vi "gl_Initialise_Images.vi"() -> (3 "Live image refs":T1)   [LabVIEW 2017]
uses:
  User Interface/Queue/Live graphs queue/Typedefs/Live imaging queue element.ctl
  <vilib>/vision/Image Controls.llb/IMAQ Image.ctl
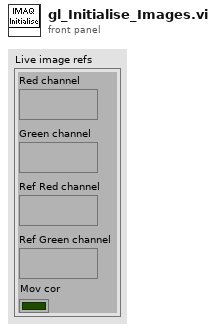
[diagram p1: front panel]
types:
  T1 = typedef "Live imaging queue element.ctl" = cluster{"Red channel":T2, "Green channel":T2, "Ref Red channel":T2, "Ref Green channel":T2, "Mov cor":bool}
  T2 = typedef "IMAQ Image.ctl" = refnum<image>
  T3 = typedef "Image Type" = u32
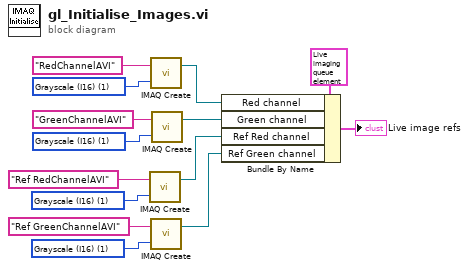
[diagram p0: block diagram]
diagram:
  w3 = T3 1 items=["Grayscale (U8)", "Grayscale (I16)", "Grayscale (SGL)", "Complex (CSG)", "RGB (U32)", "HSL (U32)", "RGB (U64)", "Grayscale (U16)"] ("Image Type")
  w6 = T3 1 items=["Grayscale (U8)", "Grayscale (I16)", "Grayscale (SGL)", "Complex (CSG)", "RGB (U32)", "HSL (U32)", "RGB (U64)", "Grayscale (U16)"] ("Image Type")
  w14 = T3 1 items=["Grayscale (U8)", "Grayscale (I16)", "Grayscale (SGL)", "Complex (CSG)", "RGB (U32)", "HSL (U32)", "RGB (U64)", "Grayscale (U16)"] ("Image Type")
  w11 = T3 1 items=["Grayscale (U8)", "Grayscale (I16)", "Grayscale (SGL)", "Complex (CSG)", "RGB (U32)", "HSL (U32)", "RGB (U64)", "Grayscale (U16)"] ("Image Type")
  n1 = call "IMAQ Create"("Image Name"="Ref RedChannelAVI", "Image Type"=w3) -> ("New Image"=w2:T2)  [unwired: 3 in, 1 out]
  n2 = call "IMAQ Create"("Image Name"="RedChannelAVI", "Image Type"=w14) -> ("New Image"=w9:T2)  [unwired: 3 in, 1 out]
  n3 = call "IMAQ Create"("Image Name"="Ref GreenChannelAVI", "Image Type"=w6) -> ("New Image"=w1:T2)  [unwired: 3 in, 1 out]
  n4 = call "IMAQ Create"("Image Name"="GreenChannelAVI", "Image Type"=w11) -> ("New Image"=w8:T2)  [unwired: 3 in, 1 out]
  n5 = Bundle By Name(cluster=T1 {"Red channel"=refnum, "Green channel"=refnum, "Ref Red channel"=refnum, "Ref Green channel"=refnum, "Mov cor"=FALSE} ("Element to queue"), "Red channel"=w9, "Green channel"=w8, "Ref Red channel"=w2, "Ref Green channel"=w1) -> (→"Live image refs":T1)
